vi "sendADCSettings.vi"(8 "error in (no error)":errorcluster, 11 "ILC in":refnum<class "ILC.lvclass">) -> (0 "error out":errorcluster, 3 "ILC out":refnum<class "ILC.lvclass">)   [LabVIEW 2015, in "ILCCommon.lvlib" / "ILC.lvclass"]
uses:
  <userlib>/Common/ILC/ILC/ILC.lvclass
  <userlib>/Common/SerialProtocols/SerialCommunicator/SerialCommunicator.lvclass
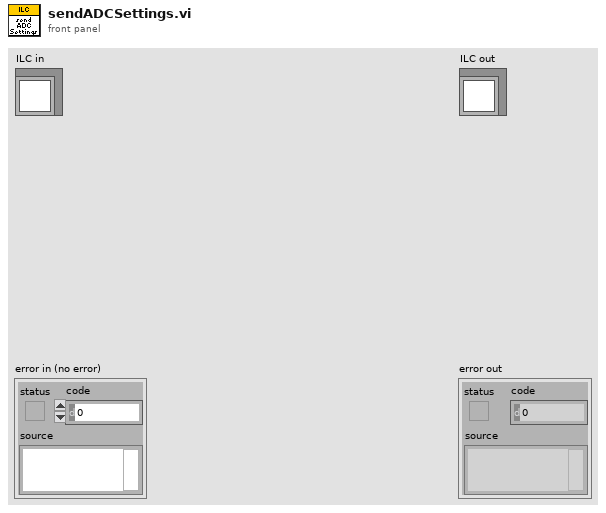
[diagram p1: front panel]
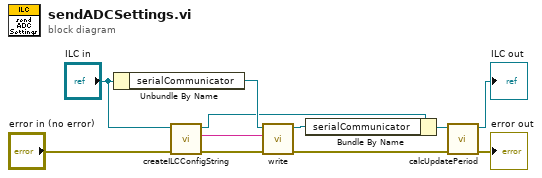
[diagram p0: block diagram]
diagram:
  n1 = Unbundle By Name("ILC in") -> ("serialCommunicator"=w10:refnum<class "SerialCommunicator.lvclass">)
  n2 = call <userlib>:"createILCConfigString.vi"("error in (no error)"="error in (no error)", "ILC in"="ILC in") -> ("error out"=w5:errorcluster, "ilcConfigurationString"=w11:string, "ILC out"=w7:refnum<class "ILC.lvclass">)  [unwired: 7 in]
  n3 = call-dynamic "write.vi"("error in (no error)"=w5, "writeString"=w11, "SerialCommunicator in"=w10) -> ("error out"=w4:errorcluster, "SerialCommunicator out"=w9:refnum<class "SerialCommunicator.lvclass">)  [unwired: 7 in]
  n4 = Bundle By Name(cluster=w7, "serialCommunicator"=w9) -> (w2:refnum<class "ILC.lvclass">)
  n5 = call <userlib>:"calcUpdatePeriod.vi"("error in (no error)"=w4, "ILC in"=w2) -> ("error out"=→"error out":errorcluster, "ILC out"=→"ILC out":refnum<class "ILC.lvclass">)  [unwired: 8 in]
